vi "_JsonFile_SetAttribute.vi"(8 "error in (no error)":errorcluster, 9 "Value":variant, 10 "Attribute":string, 11 "Json":path) -> (0 "error out":errorcluster, 3 "Json (dup)":path)   [LabVIEW 2019, in "lv-apt-json-file.lvlib"]
uses:
  lv-apt-json-file.lvlib
  <vilib>/addons/_JKI.lib/Serialization/JSON/JKI JSON Serialization.lvlib
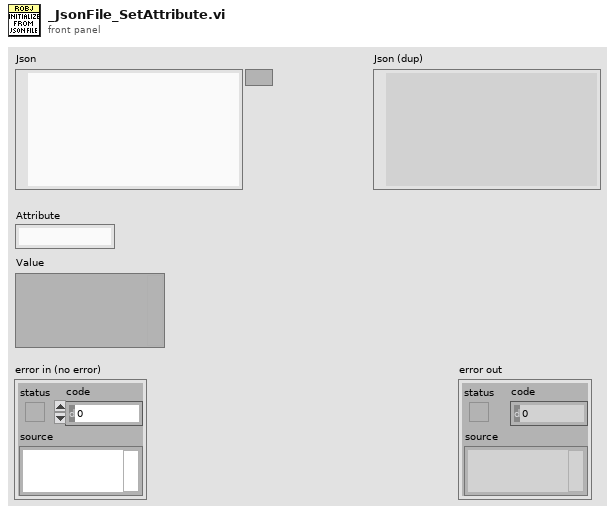
[diagram p1: front panel]
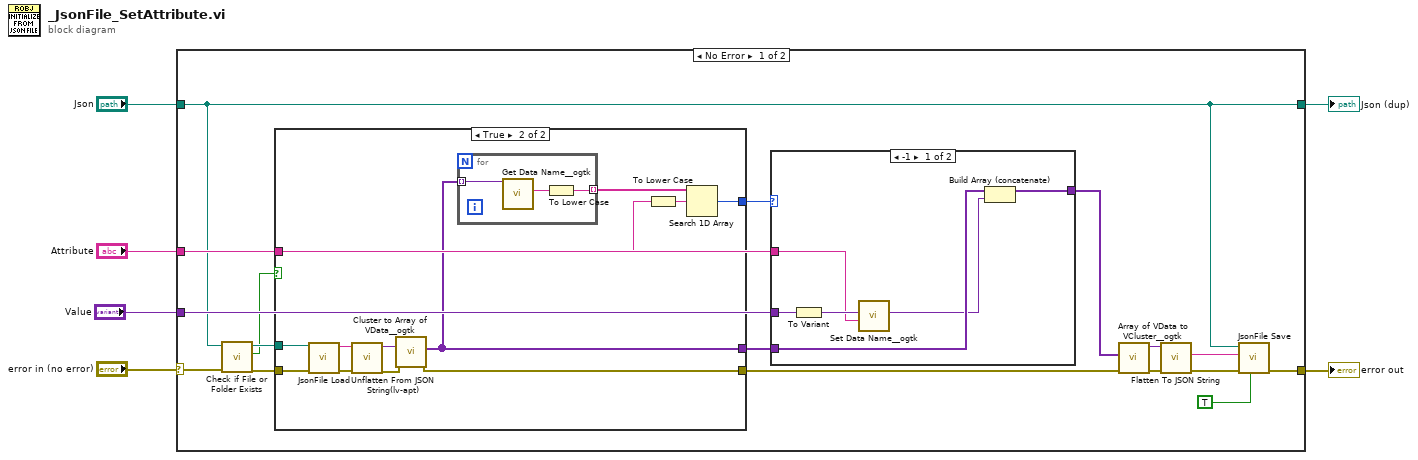
[diagram p0: block diagram]
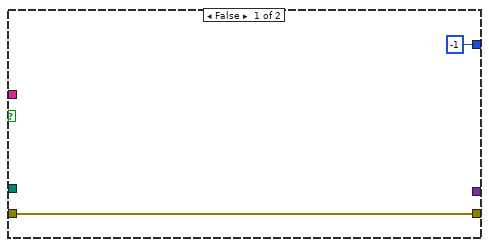
[diagram p2: hidden frame]
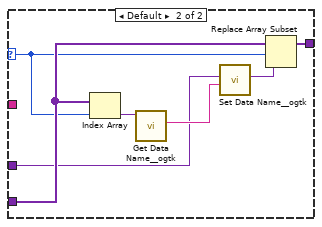
[diagram p3: hidden frame]
diagram:
  n1 = case shown="No Error" "error in (no error)" {
    selector: "error in (no error)" -> [w10 w55]
    tunnel: [w22 w55] -> w5
    tunnel: "Attribute" -> [w12 _]
    tunnel: "Value" -> [w20 _]
    tunnel: "Json" -> [w8 w54]
    tunnel: [w8 w54] -> w1
    frame No Error {
      n2 = call <vilib>:"Check if File or Folder Exists.vi"("error in (no error)"=w10, "path"=w8) -> ("error out"=w9:errorcluster, "file or folder exists?"=w7:bool, "dup path"=w11:path)  [unwired: 7 in]
      n3 = case shown="True" w7 {
        tunnel: [w25 w33] -> w23
        tunnel: [_ w31] -> w21
        tunnel: [-1 ("index of element") w29] -> w19
        tunnel: w12 -> [_ w28]
        tunnel: w11 -> [_ w27]
        tunnel: w9 -> [w25 w26]
        frame False {
        }
        frame True {
          n4 = call "JsonFile Load.vi"("error in (no error)"=w26, "Path"=w27) -> ("error out"=w35:errorcluster, "Json"=w34:string)  [unwired: 8 in]
          n5 = call "Unflatten From JSON String(lv-apt).vi"("error in (no error)"=w35, "JSON String"=w34) -> ("error out"=w37:errorcluster, "Variant"=w36:variant)  [unwired: 8 in]
          n6 = call <userlib>:"Cluster to Array of VData__ogtk.vi"("error in (no error)"=w37, "Cluster"=w36) -> ("error out"=w33:errorcluster, "Array of VData"=w31:variant[])  [unwired: 8 in]
          n7 = for {
            tunnel: w31 -> [w40] mode=indexing
            tunnel: [w39] -> w32 mode=indexing
            n8 = call <userlib>:"Get Data Name__ogtk.vi"("Data"=w40) -> ("Data Name"=w38:string)  [unwired: 8 in, 2 out]
            n9 = To Lower Case(string=w38) -> (all lower case string=w39:string)
          }
          n10 = To Lower Case(string=w28) -> (all lower case string=w30:string)
          n11 = Search 1D Array(1D array=w32, element=w30) -> (index of element=w29:i32)  [unwired: 1 in]
        }
      }
      n12 = case shown="-1" w19 {
        selector: w19 -> [_ w52]
        tunnel: w21 -> [w43 w53]
        tunnel: w20 -> [w46 w47]
        tunnel: [w42 w48] -> w18
        tunnel: w12 -> [w44 _]
        frame -1 {
          n13 = To Variant(anything=w46) -> (Variant=w45:variant)
          n14 = call <userlib>:"Set Data Name__ogtk.vi"("Data Name"=w44, "Data"=w45) -> ("Renamed Data"=w41:variant)  [unwired: 8 in, 1 out]
          n15 = Build Array (concatenate)(w43, w41) -> (w42:variant[])
        }
        frame Default {
          n16 = Index Array(array=w53, index=w52) -> (element=w50:variant)
          n17 = call <userlib>:"Get Data Name__ogtk.vi"("Data"=w50) -> ("Data Name"=w49:string)  [unwired: 8 in, 2 out]
          n18 = call <userlib>:"Set Data Name__ogtk.vi"("Data Name"=w49, "Data"=w47) -> ("Renamed Data"=w51:variant)  [unwired: 8 in, 1 out]
          n19 = Replace Array Subset(array=w53, new element=w51, index=w52) -> (w48:variant[])
        }
      }
      n20 = call <userlib>:"Array of VData to VCluster__ogtk.vi"("error in (no error)"=w23, "Array"=w18) -> ("error out"=w17:errorcluster, "VCluster"=w15:variant)  [unwired: 8 in]
      n21 = call <vilib>:"Flatten To JSON String.vi"("error in (no error)"=w17, "Variant"=w15) -> ("error out"=w16:errorcluster, "JSON String"=w14:string)  [unwired: 8 in]
      n22 = call "JsonFile Save.vi"("Pretty Print(T)"=TRUE, "error in (no error)"=w16, "JSON String"=w14, "Path"=w8) -> ("error out"=w22:errorcluster)  [unwired: 7 in]
    }
    frame Error {
    }
  }
  "error out" <- w5
  "Json (dup)" <- w1
